vi "Motor Control.vi"(0 "Kp":dbl=1.0 format="%#_13g", 1 "Kd":dbl=0.01 format="%#_13g", 2 "dt":dbl=0.001 format="%#_13g", 3 "thetad":dbl[](array[numeric])=[0.002, 0.007, 0.0], 4 "thetac":dbl[](array[numeric])=[0.0, 0.0, 0.0], 5 "e":dbl[](array[numeric])=[0.0, 0.0, 0.0]) -> (18 "thetac'":dbl[](array[numeric])=[2.1999999999999998e-07, 7.700000000000001e-07, 0.0], 19 "e'":dbl[](array[numeric])=[0.002, 0.007, 0.0])   [LabVIEW 2017]
panel:
  out "MV(voltage)":dbl[](array[numeric])=[0.022, 0.07700000000000001, 0.0]
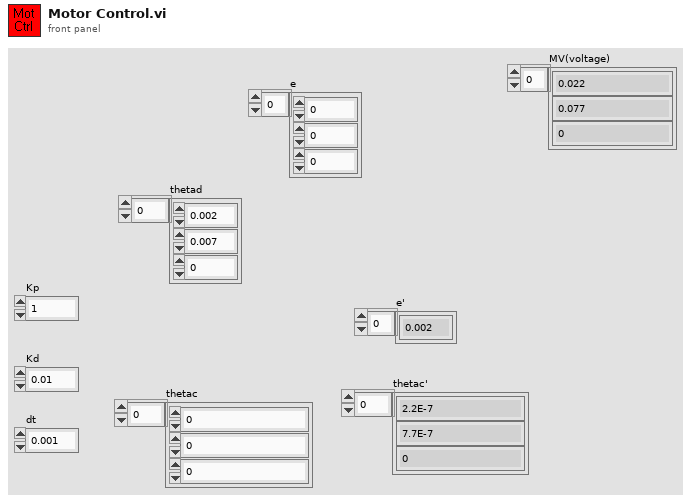
[diagram p1: front panel]
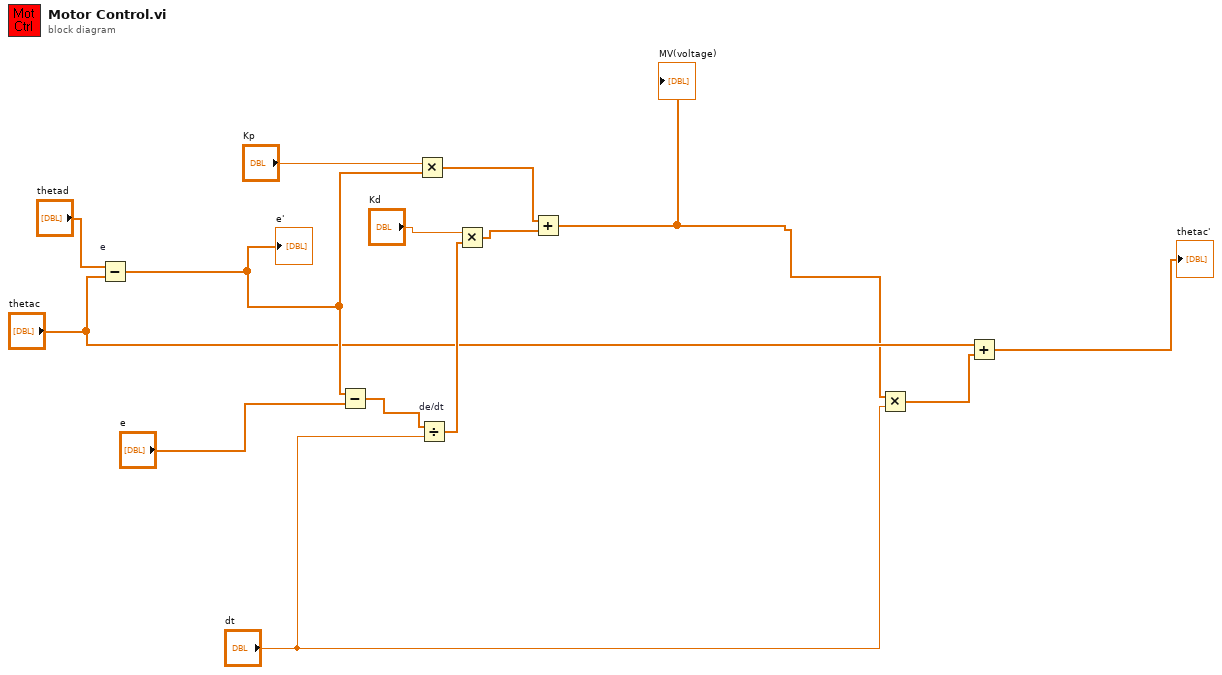
[diagram p0: block diagram]
diagram:
  n1 = Subtract "e"(x="thetad", y="thetac") -> (x-y=w11:dbl[])
  "e'" <- w11
  n2 = Subtract(x=w11, y="e") -> (x-y=w13:dbl[])
  n3 = Multiply(x="Kp", y=w11) -> (x*y=w10:dbl[])
  n4 = Divide "de/dt"(x=w13, y="dt") -> (x/y=w8:dbl[])
  n5 = Multiply(x="Kd", y=w8) -> (x*y=w7:dbl[])
  n6 = Add(x=w10, y=w7) -> (x+y=w1:dbl[])
  "MV(voltage)" <- w1
  n7 = Multiply(x=w1, y="dt") -> (x*y=w4:dbl[])
  n8 = Add(x="thetac", y=w4) -> (x+y=→"thetac'":dbl[])
